vi "ScanMode_SLM.vi"() -> ()   [LabVIEW 2014]
uses:
  Controls/Scan_SLM.ctl
  Controls/MetricControl_SLM.ctl
  Controls/Scan Metric_SLM.ctl
  Controls/ScanEngineState_SLM.ctl
  <vilib>/Analysis/6fits.llb/Curve Fitting Criteria.ctl
  <vilib>/Utility/miscctls.llb/LVPointDoubleTypeDef.ctl
  <vilib>/Analysis/NI_AALPro.lvlib
  <vilib>/gmath/NI_Gmath.lvlib
panel:
  in  "Reset":bool
  out "Image":sgl[][](graph)
  in  "Apply":bool
  in  "Find peak":bool
  in  "Cancel":bool
  in  "Metric Control":T1
  in  "stop":bool
  out "Metric Display":cluster{"Amplititude":dbl[], "Metric":dbl[]}[](graph)
  in  "Scan Control":T3 {"Mode" items=["2", "3", "4", "5", "6", "7", "8", "9", "10", "11", "12", "13", "14", "15", "16", "17", "18", "19", "20", "21", "22", "23", "24", "25", "26", "27", "28", "29", "30", "31", "32", "33", "34", "35", "36", "37"]}
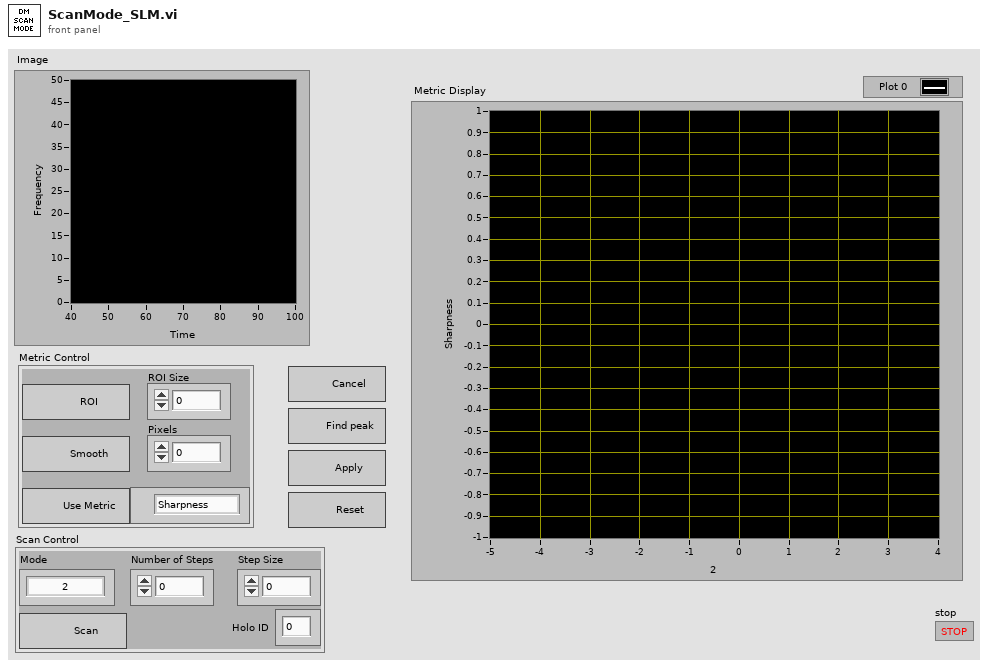
[diagram p1: front panel]
types:
  T1 = typedef "MetricControl_SLM.ctl" = cluster{"Use Metric":bool, "SLM Metric":T2, "Smooth":bool, "Pixels":dbl, "ROI":bool, "ROI Size":dbl}
  T2 = typedef "Scan Metric_SLM.ctl" = enum16{"Sharpness", "Brightness", "Combined"}
  T3 = typedef "Scan_SLM.ctl" = cluster{"Scan":bool, "Mode":u16, "Number of Steps":u8, "Step Size":dbl, "Holo ID":i32}
  T4 = typedef "ScanEngineState_SLM.ctl" = enum16{"SLM_WRITE", "IMAGE", ""}
  T5 = typedef "LVPointDoubleTypeDef.ctl" = cluster{"X":dbl, "Y":dbl}
  T6 = enum16{"Linear", "Polynomial", "Exponential", "Power"}
  T7 = typedef "Holo Settings.ctl" = cluster{"Top Hat":bool, "Modes":cluster{"Mode ID":string, "Amplititute":dbl}[], "Vortex":bool, "Clockwise":bool, "X":dbl, "Y":dbl, "Holo ON":bool, "Scan":bool}
  T8 = typedef "LVStringsAndValuesArrayTypeDef_U16.ctl" = cluster{"String":string, "Value":u16}[]
  T9 = typedef "NI_AALPro.lvlib/Curve Fitting Criteria.ctl" = u16
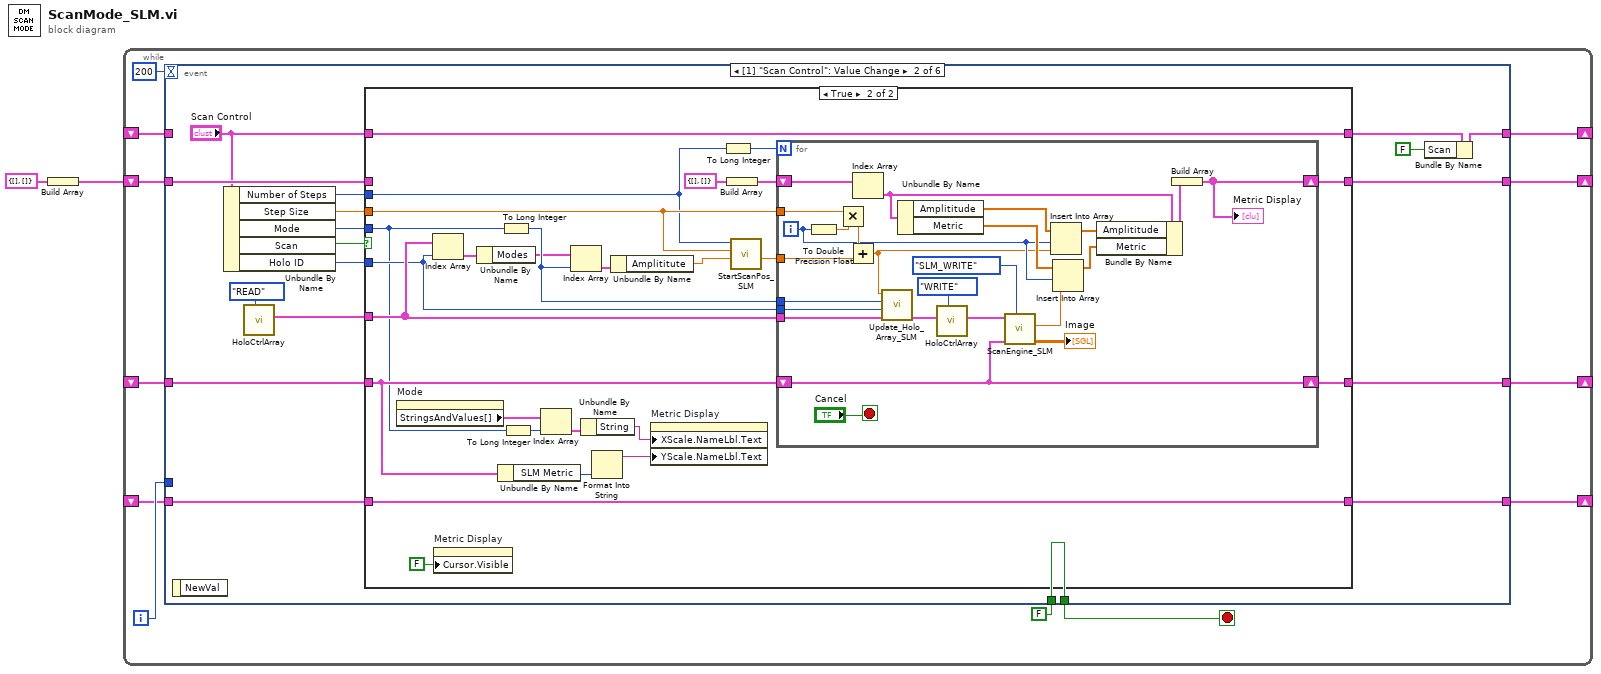
[diagram p0: block diagram]
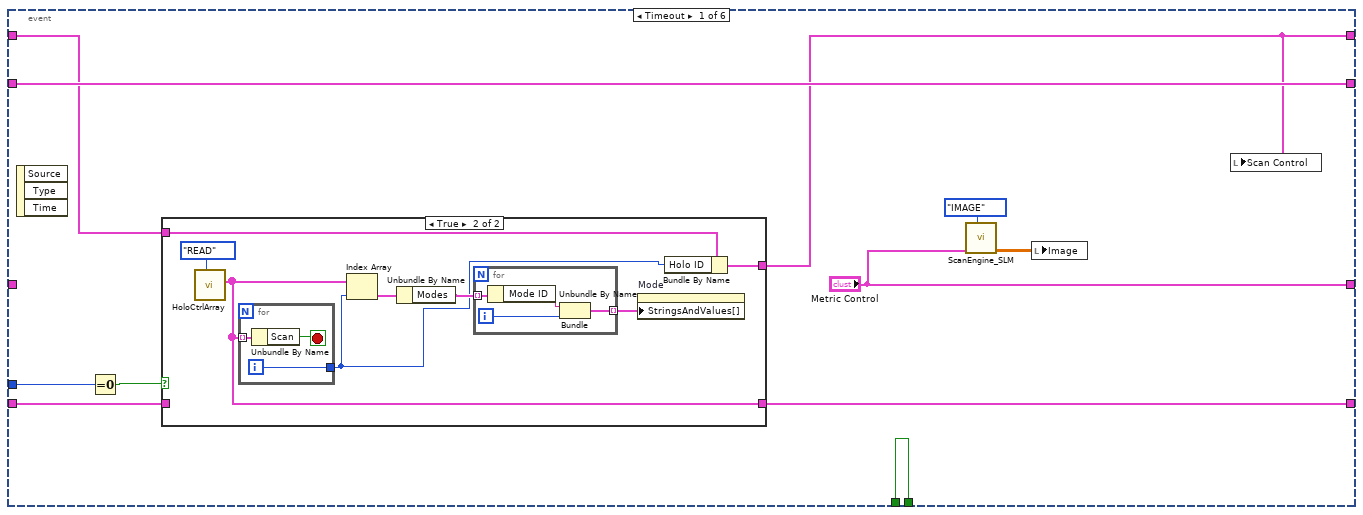
[diagram p2: hidden frame]
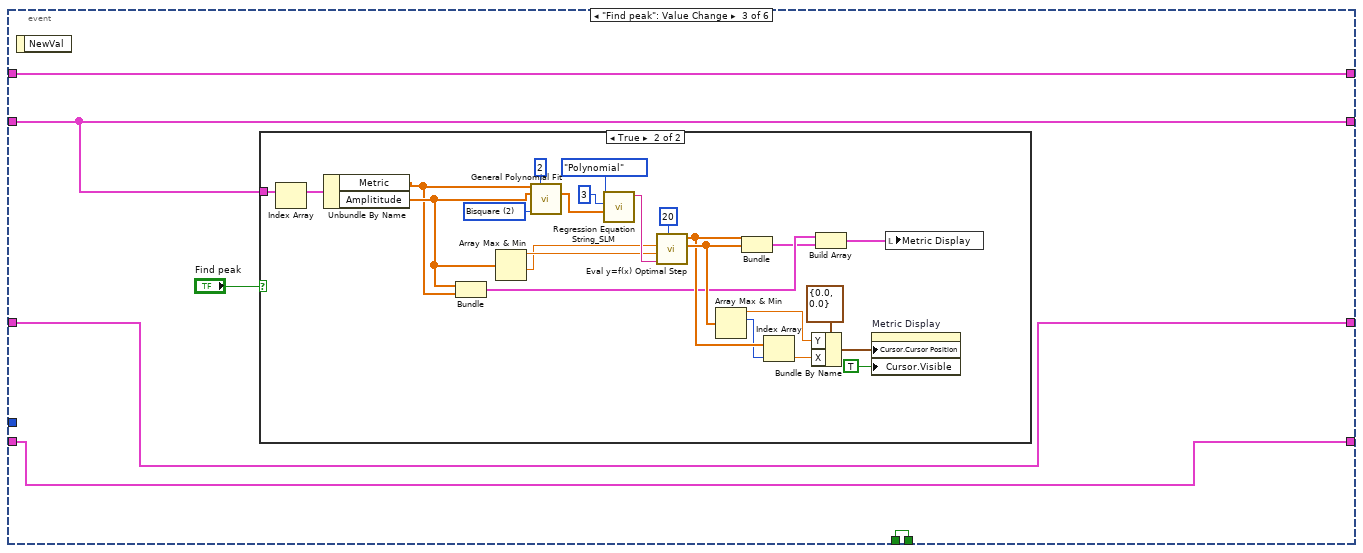
[diagram p5: hidden frame]
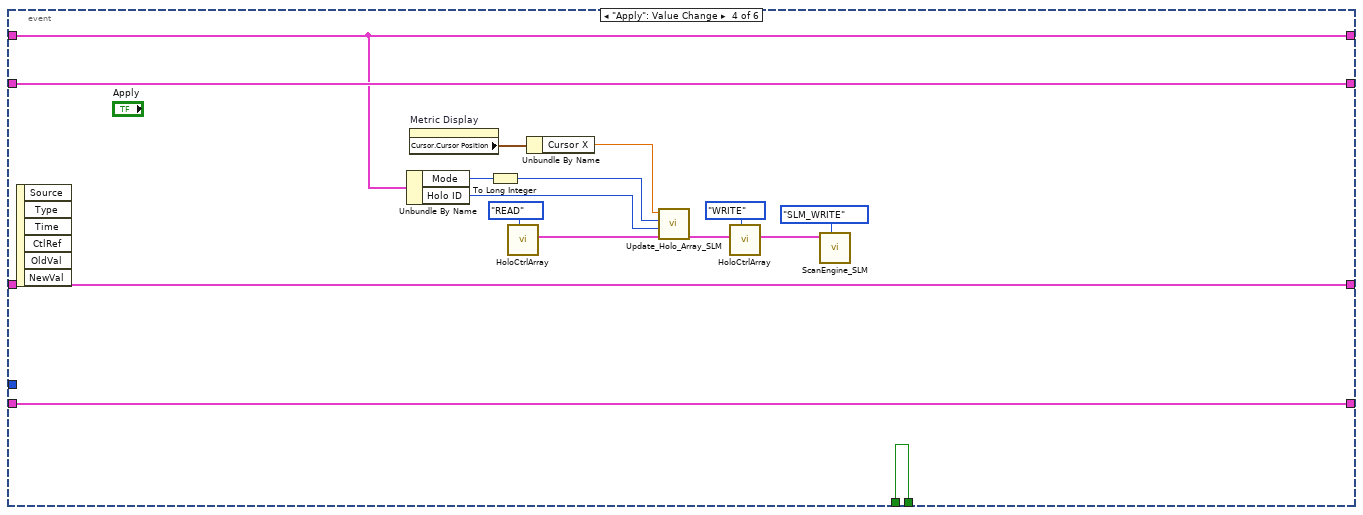
[diagram p7: hidden frame]
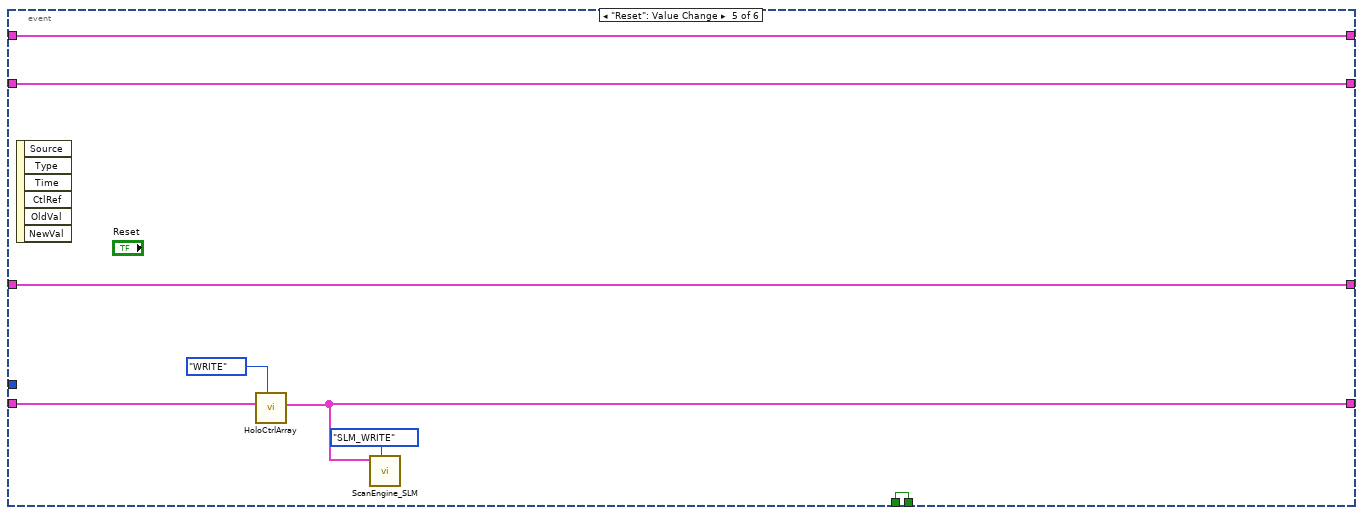
[diagram p8: hidden frame]
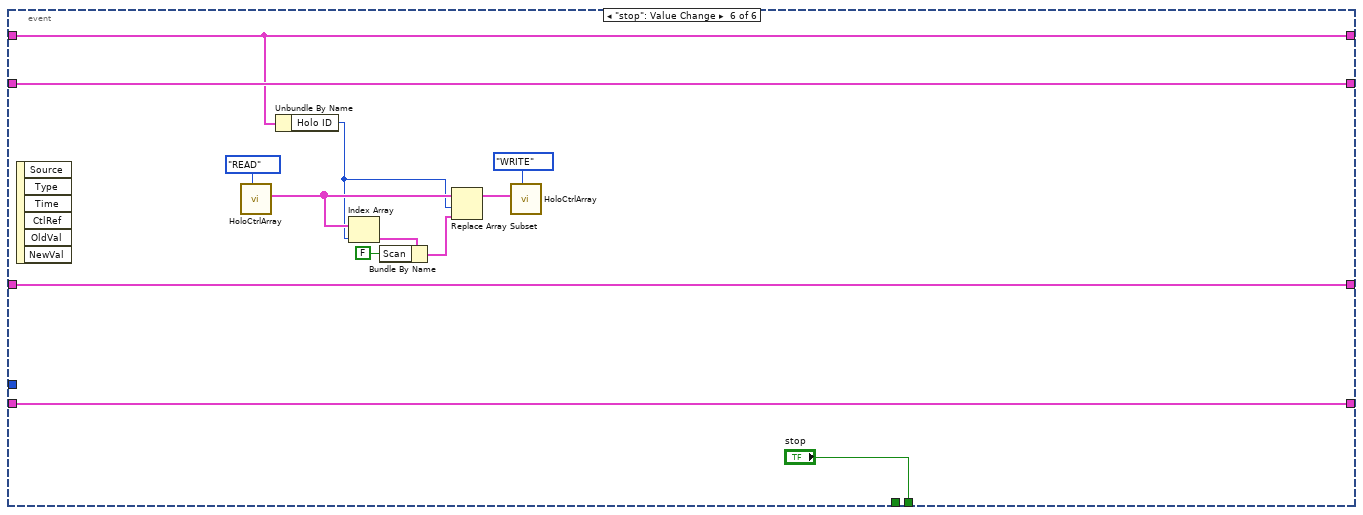
[diagram p9: hidden frame]
diagram:
  n1 = Build Array(cluster{"Amplititude":dbl[], "Metric":dbl[]} {"Amplititude"=[], "Metric"=[]} ("output cluster")) -> (w1:cluster{"Amplititude":dbl[], "Metric":dbl[]}[])
  n2 = while {
    shift-right: [w10] -> _
    shift-left: _ -> [w9]
    shift-right: [w8] -> _
    shift-left: w1 -> [w7]
    shift-right: [w5] -> _
    shift-left: _ -> [w6]
    shift-right: [w4] -> _
    shift-left: _ -> [w3]
    i -> [w11]
    stop <- w14 stop-if-true
    n3 = event shown="[1] \"Scan Control\": Value Change" {
      selector: _ -> [_ _ _ _ _ _]
      dyn-events: _ -> [_ _ _ _ _ _]
      timeout: 200 -> [_ _ _ _ _ _]
      tunnel: [w25 w58 w118 w157 w169 "stop"] -> w14
      tunnel: FALSE -> [w25 w58 w118 w157 w169 _]
      tunnel: w11 -> [w23 _ _ _ _ _]
      tunnel: [w17 w50 w121 w159 w168 w176] -> w10
      tunnel: w9 -> [w18 _ w121 w159 w168 w176]
      tunnel: [w22 w56 w120 w161 w167 w181] -> w8
      tunnel: w7 -> [w22 w54 w120 w161 w167 w181]
      tunnel: w6 -> [_ w49 w117 w156 w166 w180]
      tunnel: ["Metric Control" w45 w117 w156 w166 w180] -> w5
      tunnel: [w20 w44 w116 w146 w162 w179] -> w4
      tunnel: w3 -> [w19 w43 w116 w146 w164 w179]
      event Timeout {
        n4 = event-data() -> ()  [unwired: 1 in, 3 out]
        n5 = Equal To 0?(x=w23) -> (x = 0?=w24:bool)
        n6 = case shown="True" w24 {
          tunnel: [w27 w32] -> w20
          tunnel: w19 -> [w27 _]
          tunnel: w18 -> [w26 w31]
          tunnel: [w26 w29] -> w17
          frame False {
          }
          frame True {
            n7 = call "HoloCtrlArray.vi"("Action"=enum16{"READ", "WRITE"}."READ") -> ("Holo Array Out"=w32:T7[])  [unwired: 10 in]
            n8 = for {
              tunnel: w32 -> [w38] mode=indexing
              tunnel: [w37] -> w30
              i -> [w37]
              stop <- w36 stop-if-true
              n9 = Unbundle By Name(w38) -> ("Scan"=w36:bool)
            }
            n10 = Index Array(array=w32, index=w30) -> (element=w34:T7)
            n11 = Unbundle By Name(w34) -> ("Modes"=w33:cluster{"Mode ID":string, "Amplititute":dbl}[])
            n12 = for {
              tunnel: w33 -> [w42] mode=indexing
              tunnel: [w39] -> w28 mode=indexing
              i -> [w40]
              n13 = Unbundle By Name(w42) -> ("Mode ID"=w41:string)
              n14 = Bundle("Mode ID"=w41, w40) -> (w39:cluster{"Mode ID":string, i32})  [unwired: 1 in]
            }
            n15 = property on="Mode" class="Ring (strict)"("StringsAndValues[]"=w28) -> ()  [unwired: 2 in, 2 out]
            n16 = Bundle By Name(cluster=w31, "Holo ID"=w30) -> (w29:T3)
          }
        }
        n17 = call "ScanEngine_SLM.vi"("Action"=ScanEngineState_SLM."IMAGE", "Metric Control"="Metric Control") -> ("Metric Image"=w16:sgl[][])  [unwired: 8 in, 1 out]
        n18 = local write "Image"(w16) -> ()
        n19 = local write "Scan Control"(w17) -> ()
      }
      event Value Change {
        n20 = event-data() -> ()  [unwired: 1 in, 1 out]
        n21 = Unbundle By Name("Scan Control") -> ("Number of Steps"=w60:u8, "Step Size"=w59:dbl, "Mode"=w57:u16, "Scan"=w55:bool, "Holo ID"=w47:i32)
        n22 = call "HoloCtrlArray.vi"("Action"=enum16{"READ", "WRITE"}."READ") -> ("Holo Array Out"=w46:T7[])  [unwired: 10 in]
        n23 = case shown="True" w55 {
          tunnel: w60 -> [_ w71]
          tunnel: w59 -> [_ w90]
          tunnel: w57 -> [_ w67]
          tunnel: [w64 w79] -> w56
          tunnel: w54 -> [w64 _]
          tunnel: [w63 w83] -> w51
          tunnel: "Scan Control" -> [w63 w83]
          tunnel: w49 -> [w62 w78]
          tunnel: w47 -> [_ w74]
          tunnel: w46 -> [_ w75]
          tunnel: [w62 w73] -> w45
          tunnel: [w61 w70] -> w44
          tunnel: w43 -> [w61 w70]
          frame False {
          }
          frame True {
            n24 = property on="Mode" class="Ring (strict)"() -> ("StringsAndValues[]"=w69:T8)  [unwired: 2 in, 2 out]
            n25 = Index Array(array=w75, index=w74) -> (element=w76:T7)
            n26 = property on="Metric Display" class="XYGraph (strict)"("Cursor.Visible"=FALSE) -> ()  [unwired: 2 in, 2 out]
            n27 = Unbundle By Name(w76) -> ("Modes"=w77:cluster{"Mode ID":string, "Amplititute":dbl}[])
            n28 = Unbundle By Name(w78) -> ("SLM Metric"=w84:T2)
            n29 = To Long Integer(number=w67) -> (32bit integer=w87:i32)
            n30 = To Long Integer(number=w67) -> (32bit integer=w65:i32)
            n31 = Index Array(array=w69, index=w65) -> (element=w68:cluster{"String":string, "Value":u16})
            n32 = Index Array(array=w77, index=w87) -> (element=w88:cluster{"Mode ID":string, "Amplititute":dbl})
            n33 = Unbundle By Name(w68) -> ("String"=w66:string)
            n34 = Format Into String(w84) -> (resulting string=w85:string)  [unwired: 3 in, 1 out]
            n35 = Unbundle By Name(w88) -> ("Amplititute"=w89:dbl)
            n36 = property on="Metric Display" class="XYGraph (strict)"("XScale.NameLbl.Text"=w66, "YScale.NameLbl.Text"=w85) -> ()  [unwired: 2 in, 2 out]
            n37 = To Long Integer(number=w71) -> (32bit integer=w86:i32)
            n38 = Build Array(cluster{"Amplititude":dbl[], "Metric":dbl[]} {"Amplititude"=[], "Metric"=[]} ("output cluster")) -> (w80:cluster{"Amplititude":dbl[], "Metric":dbl[]}[])
            n39 = call "StartScanPos_SLM.vi"("Amplititute"=w89, "Step Size"=w90, "Number of Steps"=w71) -> ("Start Scan Position"=w72:dbl)  [unwired: 8 in]
            n40 = for {
              N: w86 -> [_]
              tunnel: w90 -> [w115]
              tunnel: w87 -> [w96]
              shift-right: [w102] -> w79
              shift-left: w80 -> [w111]
              tunnel: w75 -> [w94]
              tunnel: w74 -> [w95]
              shift-right: [w99] -> w73
              shift-left: w78 -> [w99]
              tunnel: w72 -> [w92]
              i -> [w108]
              stop <- "Cancel" stop-if-true
              n41 = To Double Precision Float(number=w108) -> (double precision float=w114:dbl)
              n42 = Multiply(x=w115, y=w114) -> (x*y=w113:dbl)
              n43 = Add(x=w113, y=w92) -> (x+y=w97:dbl)
              n44 = Index Array(array=w111) -> (element=w106:cluster{"Amplititude":dbl[], "Metric":dbl[]})  [unwired: 1 in]
              n45 = call "Update_Holo_Array_SLM.vi"("Holo Array In"=w94, "Holo ID"=w95, "Mode ID"=w96, "Amplititute"=w97) -> ("Update Holo Array"=w93:T7[])  [unwired: 7 in]
              n46 = Unbundle By Name(w106) -> ("Amplititude"=w110:dbl[], "Metric"=w109:dbl[])
              n47 = call "HoloCtrlArray.vi"("Action"=enum16{"READ", "WRITE"}."WRITE", "Holo Array In"=w93) -> ("Holo Array Out"=w98:T7[])  [unwired: 9 in]
              n48 = call "ScanEngine_SLM.vi"("Action"=ScanEngineState_SLM."SLM_WRITE", "Metric Control"=w99, "Holo Array In"=w98) -> ("Metric Image"=→"Image":sgl[][], "Metric Result"=w107:dbl)  [unwired: 7 in]
              n49 = Insert Into Array(array=w110, index=w108, new element=w97) -> (w105:dbl[])
              n50 = Insert Into Array(array=w109, index=w108, new element=w107) -> (w104:dbl[])
              n51 = Bundle By Name(cluster=w106, "Amplititude"=w105, "Metric"=w104) -> (w103:cluster{"Amplititude":dbl[], "Metric":dbl[]})
              n52 = Build Array(w103) -> (w102:cluster{"Amplititude":dbl[], "Metric":dbl[]}[])
              "Metric Display" <- w102
            }
          }
        }
        n53 = Bundle By Name(cluster=w51, "Scan"=FALSE) -> (w50:T3)
      }
      event "Find peak": Value Change {
        n54 = event-data() -> ()  [unwired: 1 in, 1 out]
        n55 = case shown="True" "Find peak" {
          tunnel: w120 -> [_ w126]
          frame False {
          }
          frame True {
            w145 = T9 2 items=["Least Square", "Least Absolute Residual", "Bisquare"] ("method")
            n56 = Index Array(array=w126) -> (element=w125:cluster{"Amplititude":dbl[], "Metric":dbl[]})  [unwired: 1 in]
            n57 = Unbundle By Name(w125) -> ("Metric"=w122:dbl[], "Amplititude"=w128:dbl[])
            n58 = Bundle("Amplititude"=w128, "Metric"=w122) -> (w124:cluster{"Amplititude":dbl[], "Metric":dbl[]})  [unwired: 1 in]
            n59 = Array Max & Min(array=w128) -> (max value=w138:dbl, min value=w137:dbl)  [unwired: 2 out]
            n60 = call <vilib>:"General Polynomial Fit.vi"("Y"=w122, "polynomial order"=2, "X"=w128, "method"=w145) -> ("Polynomial Coefficients"=w142:dbl[])  [unwired: 8 in, 3 out]
            n61 = call "Regression Equation String_SLM.vi"("coefficients"=w142, "precision"=3, "fit type"=T6."Polynomial") -> ("Formula"=w140:string)  [unwired: 8 in]
            n62 = call <vilib>:"Eval y=f(x) Optimal Step.vi"("number of points"=u32 20, "formula"=w140, "end"=w138, "start"=w137) -> ("Y Values"=w136:dbl[], "X Values"=w135:dbl[])  [unwired: 1 in, 2 out]
            n63 = Array Max & Min(array=w136) -> (max value=w132:dbl, max index (indices)=w134:i32)  [unwired: 2 out]
            n64 = Bundle("X Values"=w135, "Y Values"=w136) -> (w123:cluster{"X Values":dbl[], "Y Values":dbl[]})  [unwired: 1 in]
            n65 = Index Array(array=w135, index=w134) -> (element=w131:dbl)
            n66 = Bundle By Name(cluster=T5 {"X"=0.0, "Y"=0.0} ("Cursor.Cursor Position"), "Y"=w132, "X"=w131) -> (w130:T5)
            n67 = Build Array(w124, w123) -> (w127:cluster{"X Values":dbl[], "Y Values":dbl[]}[])
            n68 = property on="Metric Display" class="XYGraph (strict)"("Cursor.Cursor Position"=w130, "Cursor.Visible"=TRUE) -> ()  [unwired: 2 in, 2 out]
            n69 = local write "Metric Display"(w127) -> ()
          }
        }
      }
      event "Apply": Value Change {
        n70 = event-data() -> ()  [unwired: 1 in, 6 out]
        n71 = Unbundle By Name(w159) -> ("Mode"=w158:u16, "Holo ID"=w153:i32)
        n72 = property on="Metric Display" class="XYGraph (strict)"() -> ("Cursor.Cursor Position"=w160:T5)  [unwired: 2 in, 2 out]
        n73 = To Long Integer(number=w158) -> (32bit integer=w154:i32)
        n74 = call "HoloCtrlArray.vi"("Action"=enum16{"READ", "WRITE"}."READ") -> ("Holo Array Out"=w152:T7[])  [unwired: 10 in]
        n75 = Unbundle By Name(w160) -> ("Cursor X"=w155:dbl)
        n76 = call "Update_Holo_Array_SLM.vi"("Holo Array In"=w152, "Holo ID"=w153, "Mode ID"=w154, "Amplititute"=w155) -> ("Update Holo Array"=w149:T7[])  [unwired: 7 in]
        n77 = call "HoloCtrlArray.vi"("Action"=enum16{"READ", "WRITE"}."WRITE", "Holo Array In"=w149) -> ("Holo Array Out"=w148:T7[])  [unwired: 9 in]
        n78 = call "ScanEngine_SLM.vi"("Action"=ScanEngineState_SLM."SLM_WRITE", "Holo Array In"=w148) -> ()  [unwired: 8 in, 2 out]
      }
      event "Reset": Value Change {
        n79 = event-data() -> ()  [unwired: 1 in, 6 out]
        n80 = call "HoloCtrlArray.vi"("Action"=enum16{"READ", "WRITE"}."WRITE", "Holo Array In"=w164) -> ("Holo Array Out"=w162:T7[])  [unwired: 9 in]
        n81 = call "ScanEngine_SLM.vi"("Action"=ScanEngineState_SLM."SLM_WRITE", "Holo Array In"=w162) -> ()  [unwired: 8 in, 2 out]
      }
      event "stop": Value Change {
        n82 = event-data() -> ()  [unwired: 1 in, 6 out]
        n83 = call "HoloCtrlArray.vi"("Action"=enum16{"READ", "WRITE"}."READ") -> ("Holo Array Out"=w172:T7[])  [unwired: 10 in]
        n84 = Unbundle By Name(w176) -> ("Holo ID"=w171:i32)
        n85 = Index Array(array=w172, index=w171) -> (element=w175:T7)
        n86 = Bundle By Name(cluster=w175, "Scan"=FALSE) -> (w173:T7)
        n87 = Replace Array Subset(array=w172, new element=w173, index=w171) -> (w170:T7[])
        n88 = call "HoloCtrlArray.vi"("Action"=enum16{"READ", "WRITE"}."WRITE", "Holo Array In"=w170) -> ()  [unwired: 9 in, 1 out]
      }
    }
  }
